vi "InitDataQArrDevGen.vi"(8 "ErrorIn(No Error)":errorcluster caption="entrée d'erreur (pas d'erreur)", 10 "ArrScan list":string[](array[string]), 11 "DatArrSize":i32) -> (0 "sortie d'erreur":errorcluster, 3 "DataQ Out":refnum<queue>[](array[refnum]))   [LabVIEW 2019]
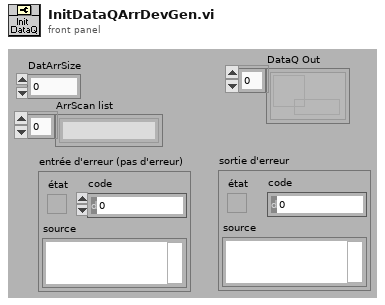
[diagram p1: front panel]
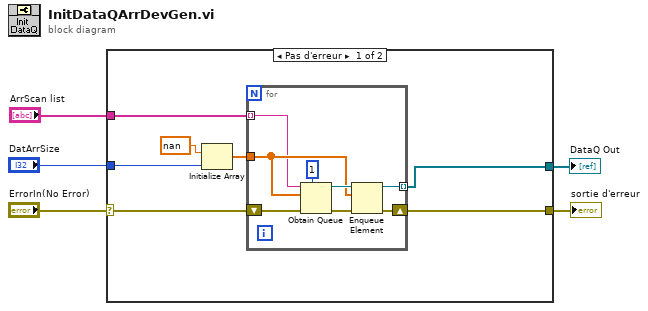
[diagram p0: block diagram]
diagram:
  n1 = case shown="Pas d'erreur" "ErrorIn(No Error)" {
    selector: "ErrorIn(No Error)" -> [w10 w21]
    tunnel: [w9 w21] -> w4
    tunnel: "DatArrSize" -> [w8 _]
    tunnel: "ArrScan list" -> [w7 _]
    tunnel: [w6 _] -> w1
    frame No Error {
      n2 = Initialize Array(nan ("élément"), w8) -> (w11:dbl[])
      n3 = for {
        tunnel: [w17] -> w6 mode=indexing
        tunnel: w11 -> [w16]
        shift-right: [w18] -> w9
        shift-left: w10 -> [w15]
        tunnel: w7 -> [w14] mode=indexing
        n4 = Obtain Queue(max queue size (-1, unlimited)=1 ("taille max de la file d'attente (-1, non limitée)"), name (unnamed)=w14, element data type=w16, error in (no error)=w15) -> (queue out=w19:refnum<queue>, error out=w20:errorcluster)  [unwired: 1 in, 1 out]
        n5 = Enqueue Element(queue=w19, element=w16, error in (no error)=w20) -> (queue out=w17:refnum<queue>, error out=w18:errorcluster)  [unwired: 1 in, 1 out]
      }
    }
    frame Error {
    }
  }
  "sortie d'erreur" <- w4
  "DataQ Out" <- w1
